vi "Post-Post Installer Build Action.vi"(11 "Folder Path":path caption="Folder Path (Empty: installer-source-distribution Build Folder)") -> ()   [LabVIEW 2020]
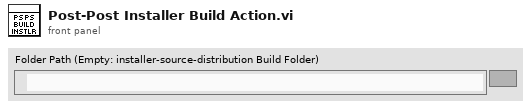
[diagram p1: front panel]
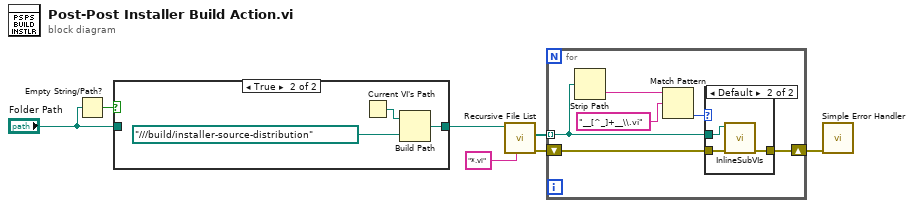
[diagram p0: block diagram]
diagram:
  n1 = Empty String/Path?(string/path="Folder Path") -> (empty?=w7:bool)
  n2 = case shown="True" w7 {
    tunnel: [w8 w9] -> w5
    tunnel: "Folder Path" -> [w8 _]
    frame False {
    }
    frame True {
      n3 = Current VI's Path() -> (path=w11:path)
      n4 = Build Path(base path=w11, name or relative path=path "../../../build/installer-source-distribution") -> (appended path=w9:path)
    }
  }
  n5 = call <vilib>:"Recursive File List.vi"("pattern"="*.vi", "Folder Path"=w5) -> ("error out"=w2:errorcluster, "All Files in Dir"=w3:path[])  [unwired: 5 in, 3 out]
  n6 = for {
    tunnel: w3 -> [w12] mode=indexing
    shift-right: [w14] -> w1
    shift-left: w2 -> [w13]
    n7 = Strip Path(path=w12) -> (name=w15:string)  [unwired: 1 out]
    n8 = Match Pattern(string=w15, regular expression="__[^_]+__\\.vi") -> (offset past match=w16:i32)  [unwired: 1 in, 3 out]
    n9 = case shown="Default" w16 {
      tunnel: [w18 w21] -> w14
      tunnel: w13 -> [w18 w20]
      tunnel: w12 -> [_ w19]
      frame -1 {
      }
      frame Default {
        n10 = call "InlineSubVIs.vi"("error in (no error)"=w20, "VI"=w19) -> ("error out"=w21:errorcluster)  [unwired: 9 in]
      }
    }
  }
  n11 = call <vilib>:"Simple Error Handler.vi"("error in (no error)"=w1) -> ()  [unwired: 4 in, 5 out]
